vi "stop_DLP_.vi"(8 "error in (no error)":errorcluster, 10 "SequenceId":u32, 11 "DeviceId":u32) -> (0 "error out":errorcluster, 2 "SequenceId Out":u32, 3 "DeviceId Out":u32)   [LabVIEW 2020]
uses:
  <vilib>/Utility/error.llb/Error Cluster From Error Code.vi
  <userlib>/alp4395/alp4395.dll
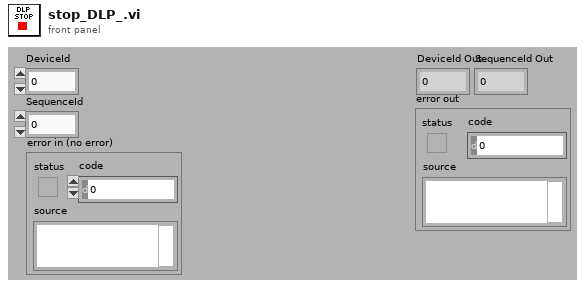
[diagram p1: front panel]
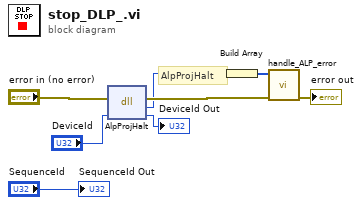
[diagram p0: block diagram]
diagram:
  # "AlpProjHalt"
  n1 = dll-call lib="C:/Program Files (x86)/National Instruments/LabVIEW 2020/user.lib/alp4395/alp4395.dll" fn="AlpProjHalt" ("Knoten zum Aufruf externer Bibliotheken")(error in="error in (no error)", "DeviceId"="DeviceId") -> (error out=w2:errorcluster, "return type"=w1:i32, "DeviceId"=→"DeviceId Out":u32)  [unwired: 2 in, 1 out]
  n2 = Build Array(w1) -> (w4:i32[])
  n3 = call "handle_ALP_error.vi"("error in"=w2, "Return Codes"=w4) -> ("error out"=→"error out":errorcluster)  [unwired: 9 in]
  "SequenceId Out" <- "SequenceId"
